vi "CheckImageQuality.vi"(8 "error in (no error)":errorcluster, 11 "Image":T1) -> (0 "error out":errorcluster, 1 "Standard  Variation":sgl, 2 "Mean Value":sgl, 3 "Within Range":bool, 4 "histogram":u32[](array[numeric]), 5 "Range":sgl, 6 "Mean +":dbl, 7 "Mean -":dbl)   [LabVIEW 2017]
uses:
  <vilib>/vision/Image Controls.llb/IMAQ Image.ctl
  <vilib>/vision/NI_Vision_Development_Module.lvlib
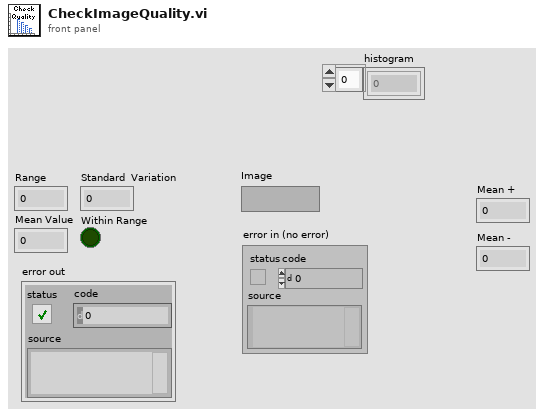
[diagram p1: front panel]
types:
  T1 = typedef "IMAQ Image.ctl" = refnum<image>
  T2 = cluster{"histogram":u32[], "Minimal Value":sgl, "Maximal Value":sgl, "Starting Value":sgl, "Interval Width":sgl, "Mean Value":sgl, "Standard  Variation":sgl, "Area (pixels)":i32}
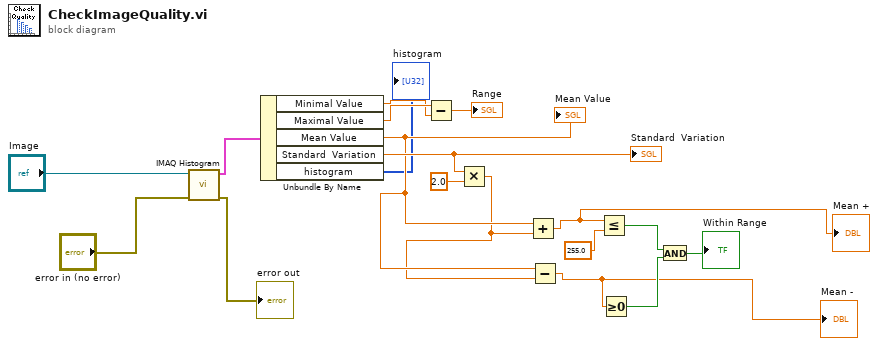
[diagram p0: block diagram]
diagram:
  n1 = call "IMAQ Histogram"("error in (no error)"="error in (no error)", "Image"="Image") -> ("error out"=→"error out":errorcluster, "Histogram Report"=w17:T2)  [unwired: 8 in]
  n2 = Unbundle By Name(w17) -> ("Minimal Value"=w15:sgl, "Maximal Value"=w16:sgl, "Mean Value"=w11:sgl, "Standard  Variation"=w12:sgl, "histogram"=→"histogram":u32[])
  "Mean Value" <- w11
  "Standard  Variation" <- w12
  n3 = Subtract(x=w16, y=w15) -> (x-y=→"Range":sgl)
  n4 = Multiply(x=w12, y=2.0) -> (x*y=w10:dbl)
  n5 = Add(x=w11, y=w10) -> (x+y=w2:dbl)
  "Mean +" <- w2
  n6 = Subtract(x=w11, y=w10) -> (x-y=w1:dbl)
  "Mean -" <- w1
  n7 = Less Or Equal?(x=w2, y=255.0) -> (x <= y?=w5:bool)
  n8 = Greater Or Equal To 0?(x=w1) -> (x >= 0?=w4:bool)
  n9 = And(x=w5, y=w4) -> (x .and. y?=→"Within Range":bool)
